vi "Backward_t.vi"(8 "error in (no error)":errorcluster, 10 "Time":dbl) -> (0 "error out":errorcluster, 2 "Done":bool)   [LabVIEW 2019]
uses:
  Timer.vi
  Simulated Robot/Simulation SubVIs/Simulation SubVIs.lvlib
panel:
  out "Diff.":dbl
  out "Left":dbl
  out "Right":dbl
  out "Diff. x Z":dbl
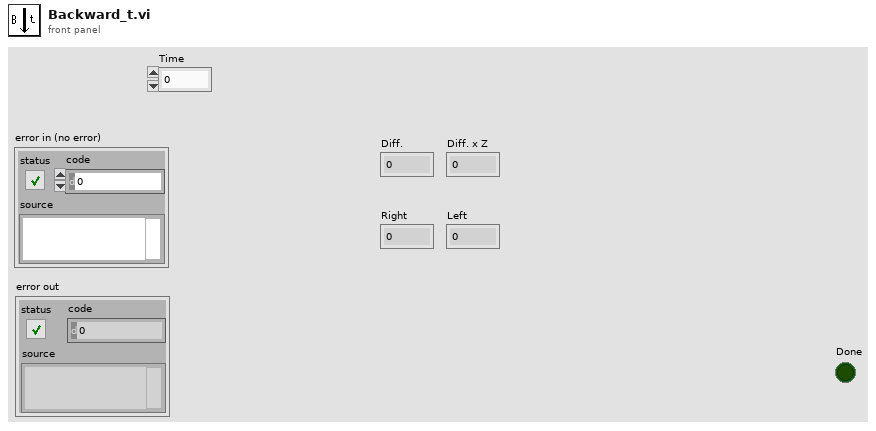
[diagram p1: front panel]
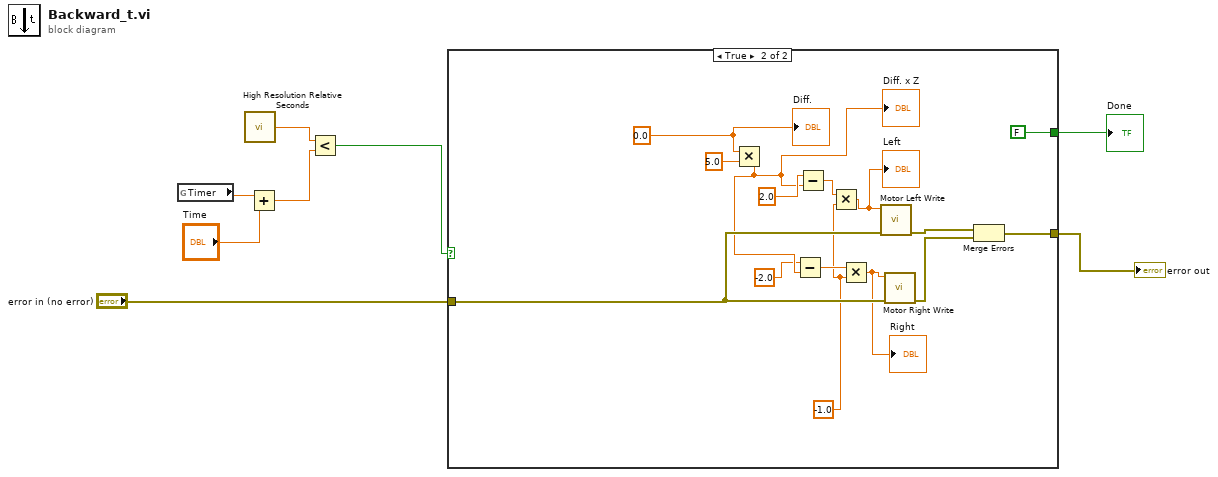
[diagram p0: block diagram]
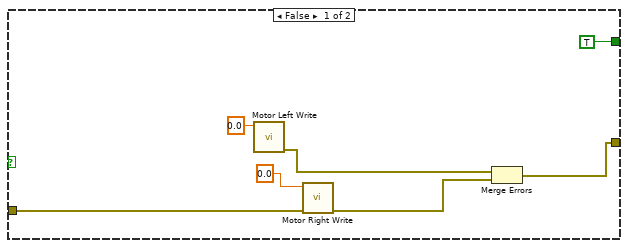
[diagram p2: hidden frame]
diagram:
  n1 = global read "Timer.vi" "Timer"() -> (w5:dbl)
  n2 = call <vilib>:"High Resolution Relative Seconds.vi"() -> ("relative seconds"=w6:dbl)
  n3 = Add(x=w5, y="Time") -> (x+y=w4:dbl)
  n4 = Less?(x=w6, y=w4) -> (x < y?=w1:bool)
  n5 = case shown="True" w1 {
    tunnel: [w11 w28] -> w8
    tunnel: "error in (no error)" -> [w10 w27]
    tunnel: [TRUE ("Done") FALSE ("Done")] -> w7
    frame False {
      n6 = call "Motor Left Write.vi"("left motor ccw velocity (rad/s)"=0.0) -> ("error out"=w15:errorcluster)  [unwired: 10 in]
      n7 = call "Motor Right Write.vi"("error in (no error)"=w10, "right motor ccw velocity (rad/s)"=0.0) -> ("error out"=w14:errorcluster)  [unwired: 9 in]
      n8 = Merge Errors(w15, w14) -> (w11:errorcluster)
    }
    frame True {
      w16 = 0.0
      w22 = -1.0
      n9 = Multiply(x=w16, y=5.0) -> (x*y=w18:dbl)
      "Diff. x Z" <- w18
      n10 = Subtract(x=-2.0 ("y"), y=w18) -> (x-y=w24:dbl)
      n11 = Subtract(x=2.0 ("left motor ccw velocity (rad/s)"), y=w18) -> (x-y=w23:dbl)
      n12 = Multiply(x=w23, y=w22) -> (x*y=w20:dbl)
      "Left" <- w20
      n13 = Multiply(x=w24, y=w22) -> (x*y=w21:dbl)
      "Right" <- w21
      n14 = call "Motor Left Write.vi"("error in (no error)"=w27, "left motor ccw velocity (rad/s)"=w20) -> ("error out"=w29:errorcluster)  [unwired: 9 in]
      n15 = call "Motor Right Write.vi"("error in (no error)"=w27, "right motor ccw velocity (rad/s)"=w21) -> ("error out"=w30:errorcluster)  [unwired: 9 in]
      n16 = Merge Errors(w29, w30) -> (w28:errorcluster)
      "Diff." <- w16
    }
  }
  "error out" <- w8
  "Done" <- w7
